vi "Untitled 5.vi"(1 "data":digitalwaveform[](array[waveform]), 2 "rate":dbl=500000.0, 4 "timeout (s)":dbl=10.0 format="%0.2f", 5 "error in":errorcluster, 7 "stop (F)":bool, 10 "device name":tag="Dev1") -> (14 "task out":refnum<k21>, 18 "stopped":bool, 19 "error out":errorcluster)   [LabVIEW 2017]
doc: "Creates, edits, and runs tasks using NI-DAQmx. Refer to the NI-DAQmx Readme for a complete listing of devices NI-DAQmx supports.\n\nWhen you place this Express VI on the block diagram, the DAQ Assistant launches to create a new task. After you create a task, you can double-click the DAQ Assistant Express VI to edit that task. For continuous measurement or generation, place a while loop around the DAQ Assistant Express VI."
uses:
  <vilib>/DAQmx/write.llb/DAQmx Write.vi
  <vilib>/DAQmx/write.llb/DAQmx Write (Digital 1D Wfm NChan NSamp).vi
  <vilib>/DAQmx/miscellaneous.llb/DAQmx Fill In Error Info.vi
  <vilib>/Waveform/DWDTOps.llb/DWDT Uncompress Digital.vi
  <vilib>/DAQmx/configure/timing.llb/DAQmx Timing (Sample Clock).vi
  <vilib>/DAQmx/create/channels.llb/DAQmx Create Channel (DO-Digital Output).vi
  <resource>/objmgr/daqmx.rc
panel:
  in  "Analog Input Sample Clock Source":tag="/Dev1/ao/SampleClock"
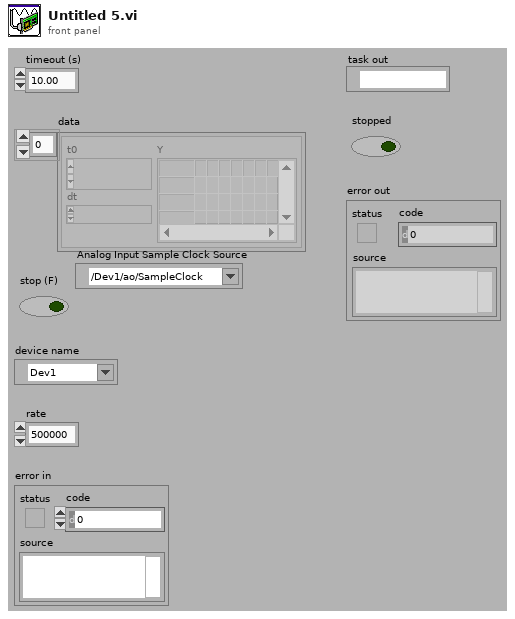
[diagram p1: front panel]
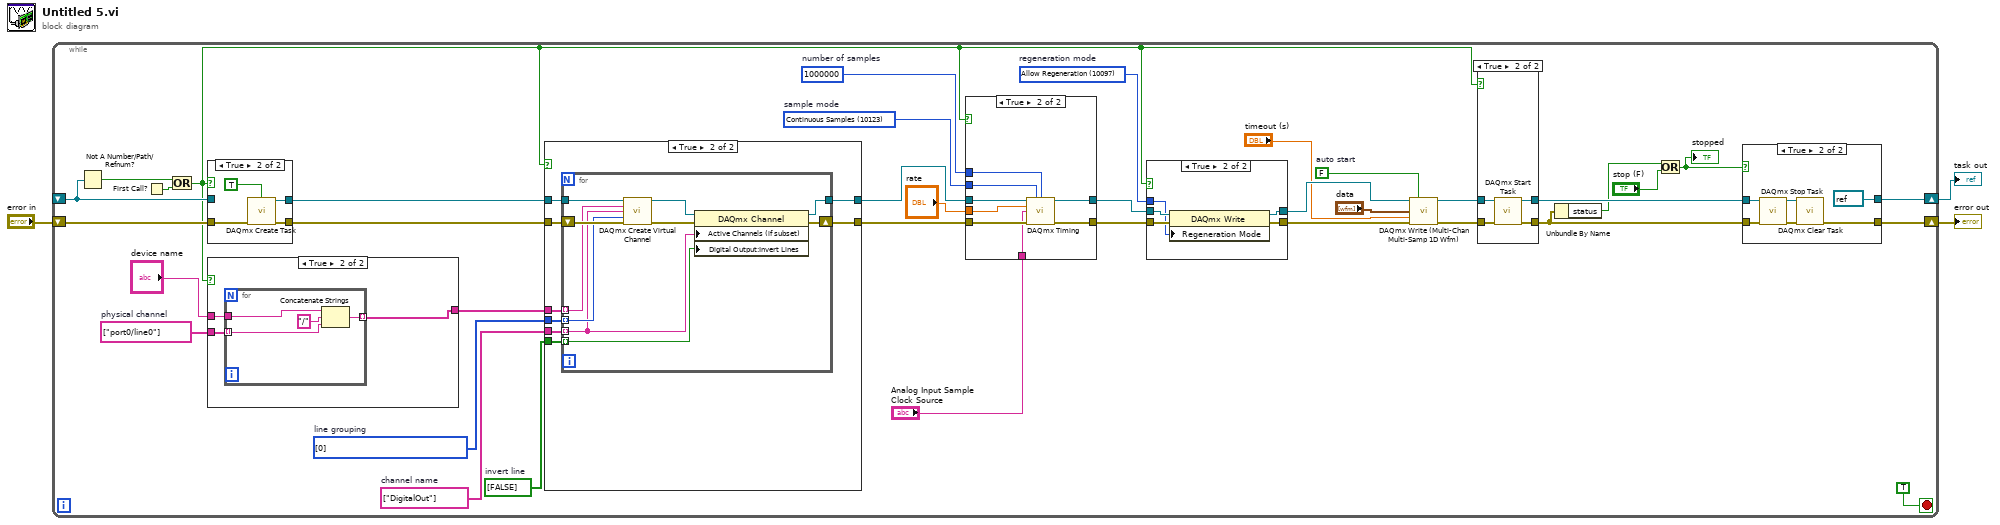
[diagram p0: block diagram]
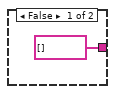
[diagram p7: hidden frame]
diagram:
  n1 = while {
    shift-right: [w11] -> w1
    shift-left: _ -> [w37]
    shift-right: [w9] -> w2
    shift-left: "error in" -> [w38]
    stop <- TRUE stop-if-true
    w17 = FALSE  # auto start
    w20 = 10097 items=["Allow Regeneration"=10097, "Do Not Allow Regeneration"=10158]  # regeneration mode
    w23 = 10123 items=["Finite Samples"=10178, "Continuous Samples"=10123, "Hardware Timed Single Point"=12522]  # sample mode
    w25 = 1000000  # number of samples
    w28 = bool[] [FALSE]  # invert line
    w29 = i32[] [0] items=["one channel for each line", "one channel for all lines"]  # line grouping
    w30 = string[] ["DigitalOut"]  # channel name
    w34 = string[] ["port0/line0"]  # physical channel
    n2 = Not A Number/Path/Refnum?(number/path/refnum=w37) -> (NaN/Path/Refnum?=w36:bool)
    n3 = First Call?() -> (First Call?: T/F=w39:bool)
    n4 = Or(x=w36, y=w39) -> (x .or. y?=w14:bool)
    n5 = case shown="True" w14 {
      tunnel: [w101 w105] -> w33
      tunnel: w37 -> [w101 _]
      tunnel: [w100 w104] -> w32
      tunnel: w38 -> [w100 w102]
      frame False {
      }
      frame True {
        n6 = call <vilib>:"DAQmx Create Task.vi"("auto cleanup"=TRUE, "error in"=w102) -> ("task out"=w105:refnum<k21>, "error out"=w104:errorcluster)  [unwired: 12 in]
      }
    }
    n7 = case shown="True" w14 {
      tunnel: [string[] [] w95] -> w31
      tunnel: "device name" -> [_ w94]
      tunnel: w34 -> [_ w93]
      frame False {
      }
      frame True {
        n8 = for {
          tunnel: [w99] -> w95 mode=indexing
          tunnel: w94 -> [w98]
          tunnel: w93 -> [w96] mode=indexing
          n9 = Concatenate Strings(w98, "/" ("string"), w96) -> (w99:string)
        }
      }
    }
    n10 = case shown="True" w14 {
      tunnel: [w73 w74] -> w27
      tunnel: w33 -> [w73 w81]
      tunnel: [w72 w79] -> w26
      tunnel: w32 -> [w72 w80]
      tunnel: w31 -> [_ w78]
      tunnel: w30 -> [_ w77]
      tunnel: w29 -> [_ w76]
      tunnel: w28 -> [_ w75]
      frame False {
      }
      frame True {
        n11 = for {
          tunnel: w81 -> [w89]
          tunnel: w78 -> [w86] mode=indexing
          tunnel: w77 -> [w84] mode=indexing
          tunnel: w76 -> [w85] mode=indexing
          tunnel: w75 -> [w83] mode=indexing
          shift-right: [w87] -> w79
          shift-left: w80 -> [w88]
          tunnel: [w82] -> w74
          n12 = call-poly <vilib>:"DAQmx Create Virtual Channel.vi"("task in"=w89, "lines"=w86, "name to assign"=w84, "line grouping"=w85, "error in"=w88) -> ("task out"=w90:refnum<k21>, "error out"=w91:errorcluster)  [unwired: 9 in]
          n13 = property class="DAQmx Channel"(reference=w90, error in=w91, "Active Channels (if subset)"=w84, "Digital Output:Invert Lines"=w83) -> (reference out=w82:refnum<k21>, error out=w87:errorcluster)
        }
      }
    }
    n14 = case shown="True" w14 {
      tunnel: [w63 w66] -> w22
      tunnel: w27 -> [w63 w69]
      tunnel: [w62 w65] -> w21
      tunnel: w26 -> [w62 w67]
      tunnel: w25 -> [_ w71]
      tunnel: w23 -> [_ w70]
      tunnel: "rate" -> [_ w68]
      tunnel: "Analog Input Sample Clock Source" -> [_ w64]
      frame False {
      }
      frame True {
        n15 = call-poly <vilib>:"DAQmx Timing.vi"("task/channels in"=w69, "sample mode"=w70, "samples per channel"=w71, "rate"=w68, "source"=w64, "error in"=w67) -> ("task out"=w66:refnum<k21>, "error out"=w65:errorcluster)  [unwired: 8 in]
      }
    }
    n16 = case shown="True" w14 {
      tunnel: w22 -> [w56 w61]
      tunnel: [w56 w60] -> w19
      tunnel: w21 -> [w55 w59]
      tunnel: [w55 w58] -> w18
      tunnel: w20 -> [_ w57]
      frame False {
      }
      frame True {
        n17 = property class="DAQmx Write"(reference=w61, error in=w59, "Regeneration Mode"=w57) -> (reference out=w60:refnum<k21>, error out=w58:errorcluster)
      }
    }
    n18 = call-poly "DAQmx Write (Multi-Chan Multi-Samp 1D Wfm).vi"("task/channels in"=w19, "auto start"=w17, "data"="data", "timeout"="timeout (s)", "error in"=w18) -> ("task out"=w13:refnum<k21>, "error out"=w12:errorcluster)  [unwired: 8 in, 1 out]
    n19 = case shown="True" w14 {
      tunnel: [w50 w53] -> w10
      tunnel: w13 -> [w50 w54]
      tunnel: [w49 w51] -> w8
      tunnel: w12 -> [w49 w52]
      frame False {
      }
      frame True {
        n20 = call <vilib>:"DAQmx Start Task.vi"("task/channels in"=w54, "error in"=w52) -> ("task out"=w53:refnum<k21>, "error out"=w51:errorcluster)  [unwired: 12 in]
      }
    }
    n21 = Unbundle By Name(w8) -> ("status"=w7:bool)
    n22 = Or(x=w7, y="stop (F)") -> (x .or. y?=w5:bool)
    "stopped" <- w5
    n23 = case shown="True" w5 {
      tunnel: [w42 refnum<k21> refnum ("task in")] -> w11
      tunnel: w10 -> [w42 w48]
      tunnel: [w41 w45] -> w9
      tunnel: w8 -> [w41 w47]
      frame False {
      }
      frame True {
        n24 = call <vilib>:"DAQmx Stop Task.vi"("task/channels in"=w48, "error in"=w47) -> ("task out"=w44:refnum<k21>, "error out"=w46:errorcluster)  [unwired: 12 in]
        n25 = call <vilib>:"DAQmx Clear Task.vi"("task in"=w44, "error in"=w46) -> ("error out"=w45:errorcluster)  [unwired: 13 in]
      }
    }
  }
  "error out" <- w2
  "task out" <- w1
